vi "SETPORT.vi"(8 "error in (no error)":errorcluster, 9 "Valor":string, 10 "Port":dbl, 11 "Arduino in":refnum<class "Arduino.lvclass">) -> (0 "error out":errorcluster, 3 "Arduino out":refnum<class "Arduino.lvclass">)   [LabVIEW 2019, in "Arduino.lvclass"]
uses:
  Arduino.lvclass
  Arduino.lvclass/Arduino.ctl
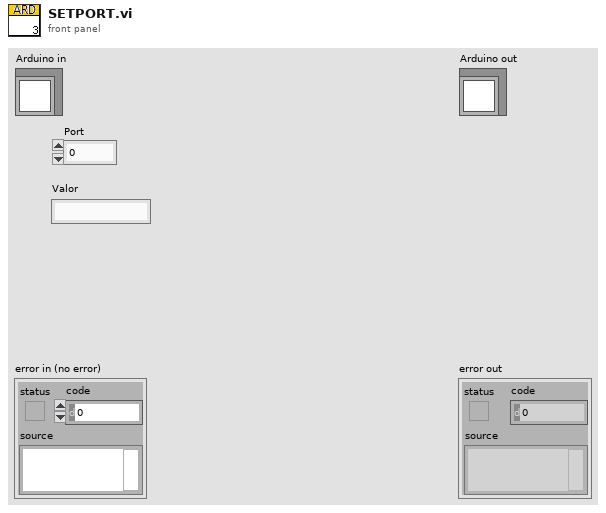
[diagram p1: front panel]
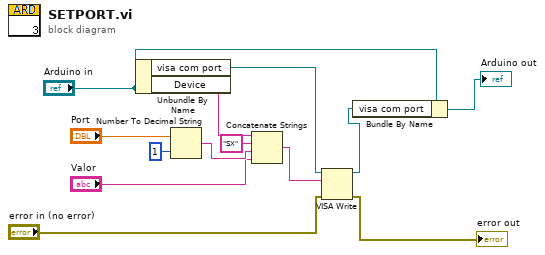
[diagram p0: block diagram]
diagram:
  n1 = Unbundle By Name("Arduino in") -> ("visa com port"=w8:refnum<visa-resource-name>, "Device"=w9:string)
  n2 = Number To Decimal String(number="Port", width (-)=i16 1) -> (decimal integer string=w5:string)
  n3 = Concatenate Strings(w9, "SX" ("string"), w5, "Valor") -> (w1:string)
  n4 = VISA Write(VISA resource name=w8, write buffer=w1, error in (no error)="error in (no error)") -> (VISA resource name out=w7:refnum<visa-resource-name>, error out=→"error out":errorcluster)  [unwired: 1 out]
  n5 = Bundle By Name(cluster="Arduino in", "visa com port"=w7) -> (→"Arduino out":refnum<class "Arduino.lvclass">)
